vi "Translator.Control.Fglb.vi"(7 "Action":T3, 8 "error in (no error)":errorcluster, 10 "Controls in":T1[](array[typedef]), 11 "VI ref in":refnum<vi>) -> (0 "error out":errorcluster, 2 "Controls out":T1[](array[typedef]), 3 "VI ref out":refnum<vi>)   [LabVIEW 2019, in "Tools.lvlib"]
uses:
  Tools.lvlib
  Translator.ControlData.ctl
  Translator.ControlTypes.ctl
  Translator.Control.Fglb.Action.vi
  Translator.Global.vi
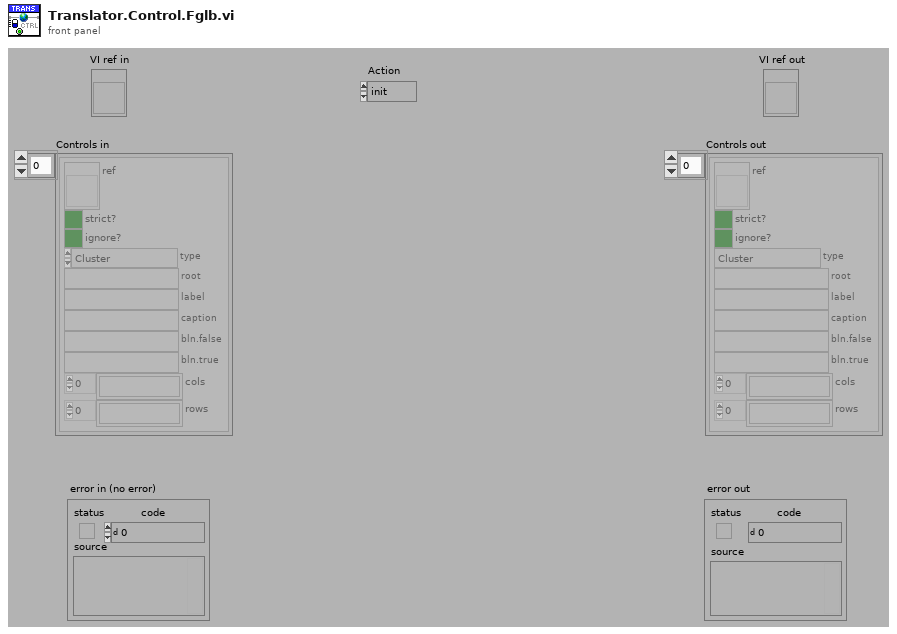
[diagram p1: front panel]
types:
  T1 = typedef "Tools.lvlib/Translator.ControlData.ctl" = cluster{"ref":refnum<vi>, "strict?":bool, "ignore?":bool, "type":T2, "root":string, "label":string, "caption":string, "bln.false":string, "bln.true":string, "cols":string[], "rows":string[]}
  T2 = typedef "Tools.lvlib/Translator.ControlTypes.ctl" = enum16{"Cluster", "Array", "Boolean", "Ring", "String", "Tab", "Listbox", "Multicolumn listbox", "Table", "Other"}
  T3 = typedef "Tools.lvlib/Translator.Control.Fglb.Action.vi" = enum16{"init", "set", "get", "clear"}
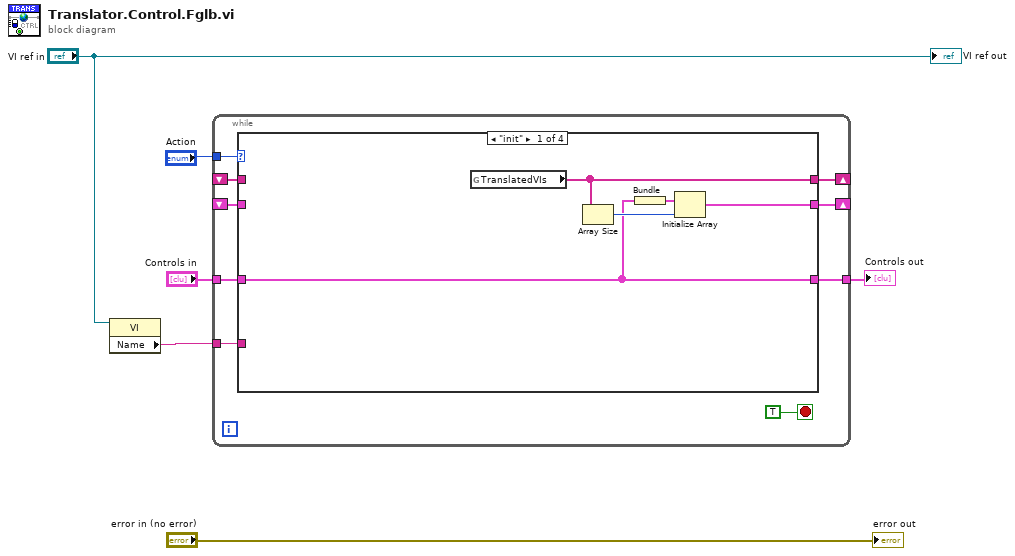
[diagram p0: block diagram]
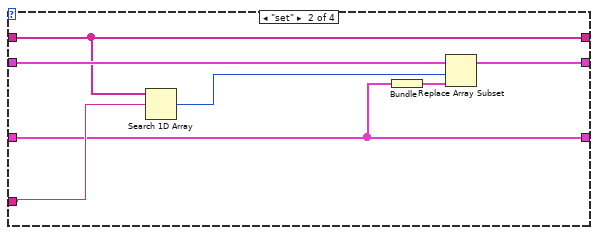
[diagram p2: hidden frame]
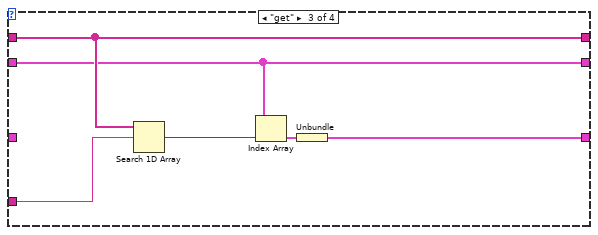
[diagram p3: hidden frame]
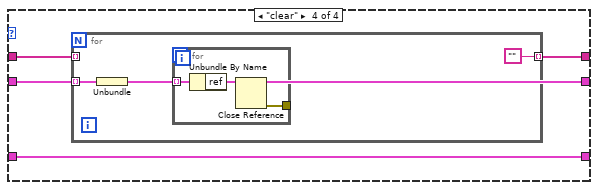
[diagram p4: hidden frame]
diagram:
  n1 = property class="VI"(reference="VI ref in") -> ("Name"=w1:string)  [unwired: 1 in, 2 out]
  n2 = while {
    tunnel: "Action" -> [w14]
    tunnel: "Controls in" -> [w13]
    tunnel: [w12] -> w3
    tunnel: w1 -> [w11]
    shift-right: [w10] -> _
    shift-left: _ -> [w9]
    shift-right: [w7] -> _
    shift-left: _ -> [w8]
    stop <- TRUE stop-if-true
    n3 = case shown="\"init\"" w14 {
      tunnel: [w18 w21 w29 w34] -> w12
      tunnel: w13 -> [w18 w21 _ w34]
      tunnel: w11 -> [_ w25 w33 _]
      tunnel: [w20 w24 w32 w36] -> w10
      tunnel: w9 -> [_ w24 w32 w37]
      tunnel: w8 -> [_ w27 w31 w35]
      tunnel: [w16 w26 w31 w35] -> w7
      frame "init" {
        n4 = global read "Translator.Global.vi" "TranslatedVIs"() -> (w20:string[])
        n5 = Array Size(array=w20) -> (size(s)=w19:i32)
        n6 = Bundle("Controls in"=w18) -> (w17:cluster{"Controls in":T1[]})  [unwired: 1 in]
        n7 = Initialize Array(w17, w19) -> (w16:cluster{"Controls in":T1[]}[])
      }
      frame "set" {
        n8 = Search 1D Array(1D array=w24, element=w25) -> (index of element=w23:i32)  [unwired: 1 in]
        n9 = Bundle("Controls in"=w21) -> (w22:cluster{"Controls in":T1[]})  [unwired: 1 in]
        n10 = Replace Array Subset(array=w27, new element=w22, index=w23) -> (w26:cluster{"Controls in":T1[]}[])
      }
      frame "get" {
        n11 = Search 1D Array(1D array=w32, element=w33) -> (index of element=w28:i32)  [unwired: 1 in]
        n12 = Index Array(array=w31, index=w28) -> (element=w30:cluster{"Controls in":T1[]})
        n13 = Unbundle(w30) -> ("Controls in"=w29:T1[])
      }
      frame "clear" {
        n14 = for {
          tunnel: w35 -> [w40] mode=indexing
          tunnel: w37 -> [_] mode=indexing
          tunnel: [""] -> w36 mode=indexing
          n15 = Unbundle(w40) -> ("Controls in"=w39:T1[])
          n16 = for {
            tunnel: w39 -> [w43] mode=indexing
            tunnel: [w41] -> _
            n17 = Unbundle By Name(w43) -> ("ref"=w42:refnum<vi>)
            n18 = Close Reference(reference=w42) -> (error out=w41:errorcluster)  [unwired: 1 in]
          }
        }
      }
    }
  }
  "Controls out" <- w3
  "error out" <- "error in (no error)"
  "VI ref out" <- "VI ref in"
